vi "Unmarshal.vi"(8 "error in (no error)":errorcluster, 10 "Buffer":u8[](array[numeric]), 11 "int32 in":refnum<class "string.lvclass">) -> (0 "error out":errorcluster, 2 "Buffer Count":i32=8, 3 "int32 out":refnum<class "string.lvclass">)   [LabVIEW 2020, in "Protobuf RAW.lvlib" / "string.lvclass"]
uses:
  string.lvclass
  string.lvclass/string.ctl
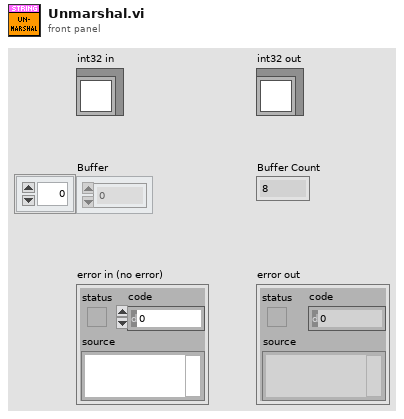
[diagram p1: front panel]
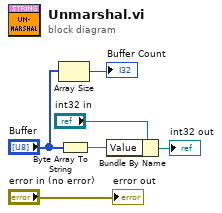
[diagram p0: block diagram]
diagram:
  n1 = Array Size(array="Buffer") -> (size(s)=→"Buffer Count":i32)
  n2 = Byte Array To String(unsigned byte array="Buffer") -> (string=w3:string)
  n3 = Bundle By Name(cluster="int32 in", "Value"=w3) -> (→"int32 out":refnum<class "string.lvclass">)
  "error out" <- "error in (no error)"
